vi "Write Instrument Driver Type.vi"(8 "error in":errorcluster, 10 "Instrument Driver.lvclass":refnum<class "Instrument Driver.lvclass">, 11 "Plugin_Driver in":refnum<class "Plugin_Driver.lvclass">) -> (0 "error out":errorcluster, 3 "Plugin_Driver out":refnum<class "Plugin_Driver.lvclass">)   [LabVIEW 2020, in "Plugin.lvlib" / "Plugin_Driver.lvclass"]
doc: "Write Instrument Driver Type"
uses:
  Plugin_Driver.lvclass
  Drivers/Instrument Driver/Instrument Driver.lvclass
  Plugin_Driver.lvclass/Plugin_Driver.ctl
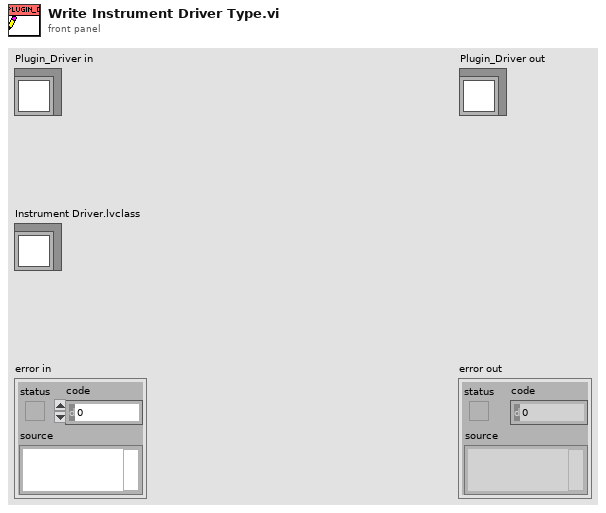
[diagram p1: front panel]
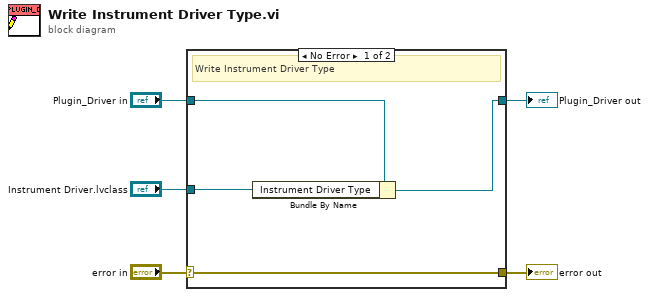
[diagram p0: block diagram]
diagram:
  n1 = case shown="No Error" "error in" {
    selector: "error in" -> [w9 w10]
    tunnel: [w9 w10] -> w4
    tunnel: [w7 w11] -> w2
    tunnel: "Plugin_Driver in" -> [w8 w11]
    tunnel: "Instrument Driver.lvclass" -> [w6 _]
    frame No Error {
      # "Write Instrument Driver Type"
      n2 = Bundle By Name(cluster=w8, "Instrument Driver Type"=w6) -> (w7:refnum<class "Plugin_Driver.lvclass">)
    }
    frame Error {
      # "Error"
    }
  }
  "error out" <- w4
  "Plugin_Driver out" <- w2
